vi "LeftRight.vi"   [LabVIEW 2017]
types:
  T1 = typedef "Command Status Info.ctl" = cluster{"Name":string, "Status":T2, "notifier out":T3}
  T2 = typedef "Completion Status.ctl" = enum16{"Successful", "Aborted", "Incomplete"}
  T3 = typedef "Completion Notifier.ctl" = refnum<notifier>
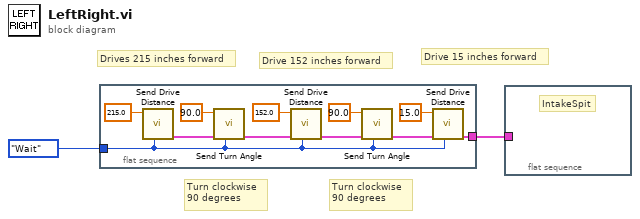
[diagram p0: block diagram]
diagram:
  # "Drive 15 inches forward"
  # "Turn clockwise\n90 degrees"
  # "Drive 152 inches forward"
  # "Turn clockwise\n90 degrees"
  # "Drives 215 inches forward"
  n1 = flat-sequence {
    tunnel: [w4] -> w1
    tunnel: enum16{"Start", "Wait"}."Wait" ("Synchronization") -> [w3]
    frame #0 {
      n2 = call "Send Drive Distance.vi"("Synchronization"=w3, "Target Distance"=215.0) -> ("Command Info Out"=w8:T1)  [unwired: 8 in, 1 out]
      n3 = call "Send Turn Angle.vi"("Synchronization"=w3, "Command Info In"=w8, "Target Angle"=90.0) -> ("Command Info Out"=w7:T1)  [unwired: 7 in, 1 out]
      n4 = call "Send Drive Distance.vi"("Synchronization"=w3, "Command Info In"=w7, "Target Distance"=152.0) -> ("Command Info Out"=w6:T1)  [unwired: 7 in, 1 out]
      n5 = call "Send Turn Angle.vi"("Synchronization"=w3, "Command Info In"=w6, "Target Angle"=90.0) -> ("Command Info Out"=w5:T1)  [unwired: 7 in, 1 out]
      n6 = call "Send Drive Distance.vi"("Synchronization"=w3, "Command Info In"=w5, "Target Distance"=15.0) -> ("Command Info Out"=w4:T1)  [unwired: 7 in, 1 out]
    }
  }
  n7 = flat-sequence {
    tunnel: w1 -> [_]
    frame #0 {
      # "IntakeSpit"
    }
  }
